vi "PSD.vi"(11 "Array in":dbl[](array[numeric])) -> (3 "Array out":dbl[](array[numeric]))   [LabVIEW 2012]
uses:
  <vilib>/Analysis/4window.llb/Hanning Window (DBL).vi
  <vilib>/Analysis/2dsp.llb/Real FFT.vi
  <vilib>/Analysis/NI_AALPro.lvlib
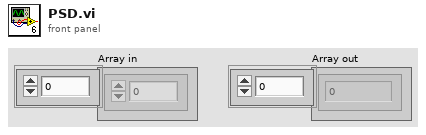
[diagram p1: front panel]
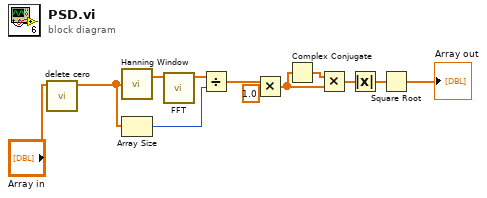
[diagram p0: block diagram]
diagram:
  n1 = call "delete cero.vi"("Array in"="Array in") -> ("Array 3"=w7:dbl[])  [unwired: 10 in]
  n2 = call-poly <vilib>:"Hanning Window.vi"("X"=w7) -> ("Windowed X"=w1:dbl[])  [unwired: 1 out]
  n3 = Array Size(array=w7) -> (size(s)=w8:i32)
  n4 = call-poly <vilib>:"FFT.vi"("X"=w1) -> ("FFT {X}"=w11:cdb[])  [unwired: 9 in, 1 out]
  n5 = Divide(x=w11, y=w8) -> (x/y=w9:cdb[])
  n6 = Multiply(x=w9, y=1.0) -> (x*y=w12:cdb[])
  n7 = Complex Conjugate(1:w12) -> (0:w2:cdb[])
  n8 = Multiply(x=w2, y=w12) -> (x*y=w3:cdb[])
  n9 = Absolute Value(x=w3) -> (abs(x)=w4:dbl[])
  n10 = Square Root(x=w4) -> (sqrt(x)=→"Array out":dbl[])
